vi "ZMC Up3File To Mem.vi"(0 "handle":u32, 1 "puifilesize":u32, 5 "pbuffer":string, 7 "buffsize":u32, 9 "pfilenameinControl":string, 11 "error in (no error)":errorcluster caption="错误输入（无错误）") -> (3 "puifilesize out":u32, 4 "handle out":u32, 6 "pbuffer out":string, 8 "function return":i32, 15 "error out":errorcluster caption="错误输出")   [LabVIEW 2015, in "zauxdll.lvlib"]
doc: "int32 __stdcall ZMC_Up3FileToMem(ZMC_HANDLE handle, char* pbuffer, uint32 buffsize, const char* pfilenameinControl, uint32* puifilesize);"
uses:
  zauxdll.lvlib
  zmotion.dll
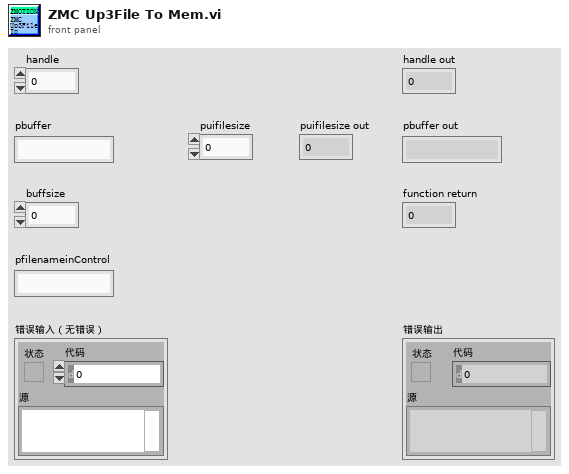
[diagram p1: front panel]
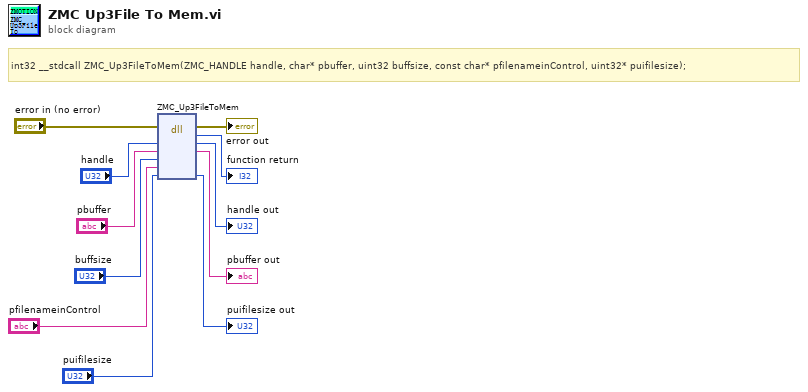
[diagram p0: block diagram]
diagram:
  # "int32 __stdcall ZMC_Up3FileToMem(ZMC_HANDLE handle, char* pbuffer, uint32 buffsize, const char* pfilenameinControl, uint32* puifilesize);"
  n1 = dll-call lib="C:/Users/VIC/Desktop/GOGORO_SA/system/LLB/zmotion/zaux/zmotion.*" fn="ZMC_Up3FileToMem"(error in="error in (no error)", "handle"="handle", "pbuffer"="pbuffer", "buffsize"="buffsize", "pfilenameinControl"="pfilenameinControl", "puifilesize"="puifilesize") -> (error out=→"error out":errorcluster, →"function return":i32, "handle"=→"handle out":u32, "pbuffer"=→"pbuffer out":string, "puifilesize"=→"puifilesize out":u32)  [unwired: 4 in, 1 out]
